vi "Derivative Control Points.vi"(11 "ctrl points":cluster{dbl, dbl}[](array[cluster])) -> (3 "d ctrl pts":cluster{dbl, dbl}[](array[cluster]))   [LabVIEW 2019]
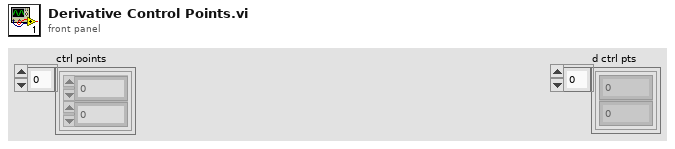
[diagram p1: front panel]
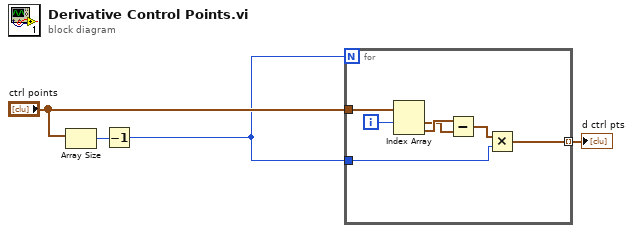
[diagram p0: block diagram]
diagram:
  n1 = Array Size(array="ctrl points") -> (size(s)=w4:i32)
  n2 = Decrement(x=w4) -> (x-1=w1:i32)
  n3 = for {
    N: w1 -> [_]
    tunnel: "ctrl points" -> [w11]
    tunnel: w1 -> [w6]
    tunnel: [w5] -> w2 mode=indexing
    i -> [w10]
    n4 = Index Array(array=w11, index #1=w10) -> (element #1=w8:cluster{dbl, dbl}, element #2=w9:cluster{dbl, dbl})  [unwired: 1 in]
    n5 = Subtract(x=w9, y=w8) -> (x-y=w7:cluster{dbl, dbl})
    n6 = Multiply(x=w7, y=w6) -> (x*y=w5:cluster{dbl, dbl})
  }
  "d ctrl pts" <- w2
